vi "Type Color.vi"(8 "error in (no error)":errorcluster, 11 "MySquare in":refnum<class "MySquare.lvclass">) -> (0 "error out":errorcluster, 2 "Type Color":u32(colorbox)=9868950, 3 "MySquare out":refnum<class "MySquare.lvclass">)   [LabVIEW 2020, in "Clones.lvlib" / "MySquare.lvclass"]
uses:
  MySquare.lvclass
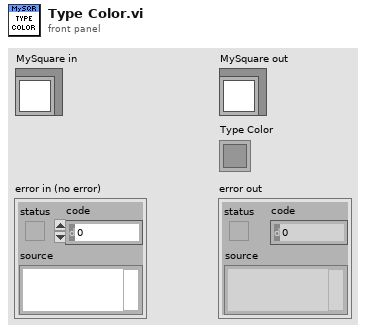
[diagram p1: front panel]
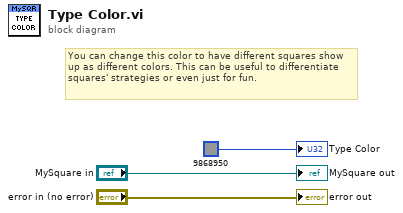
[diagram p0: block diagram]
diagram:
  # "You can change this color to have different squares show up as different colors. This can be useful to differentiate squares' strategies or even just for fun."
  "error out" <- "error in (no error)"
  "MySquare out" <- "MySquare in"
  "Type Color" <- u32 9868950 ("Type Color")
